vi "Get Transformation Matrix.vi"(9 "Z Axis Rotate Angle":sgl, 10 "Y Axis Rotate Angle":sgl, 11 "Quiver Vector":cluster{"X":sgl, "Y":sgl, "Z":sgl}) -> (1 "Transtlate to Quiver Vertex":sgl[][](array[numeric])=[[1.0, 0.0, 0.0, 0.0], [0.0, 1.0, 0.0, 0.0], [0.0, 0.0, 1.0, 0.0], [0.0, 0.0, 0.0, 1.0]], 2 "Rotate by Z Axis":sgl[][](array[numeric])=[[1.0, 0.0, 0.0, 0.0], [0.0, 1.0, 0.0, 0.0], [0.0, 0.0, 1.0, 0.0], [0.0, 0.0, 0.0, 1.0]], 3 "Rotate by Y Axis":sgl[][](array[numeric])=[[1.0, 0.0, 0.0, 0.0], [0.0, 1.0, 0.0, 0.0], [0.0, 0.0, 1.0, 0.0], [0.0, 0.0, 0.0, 1.0]])   [LabVIEW 2017, in "3D Quiver.lvclass"]
uses:
  <vilib>/Math Plots/3D Math Plots/3D Quiver/3D Quiver/3D Quiver.lvclass
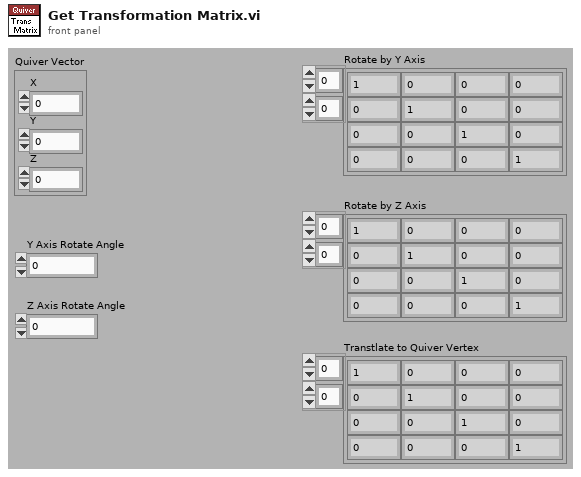
[diagram p1: front panel]
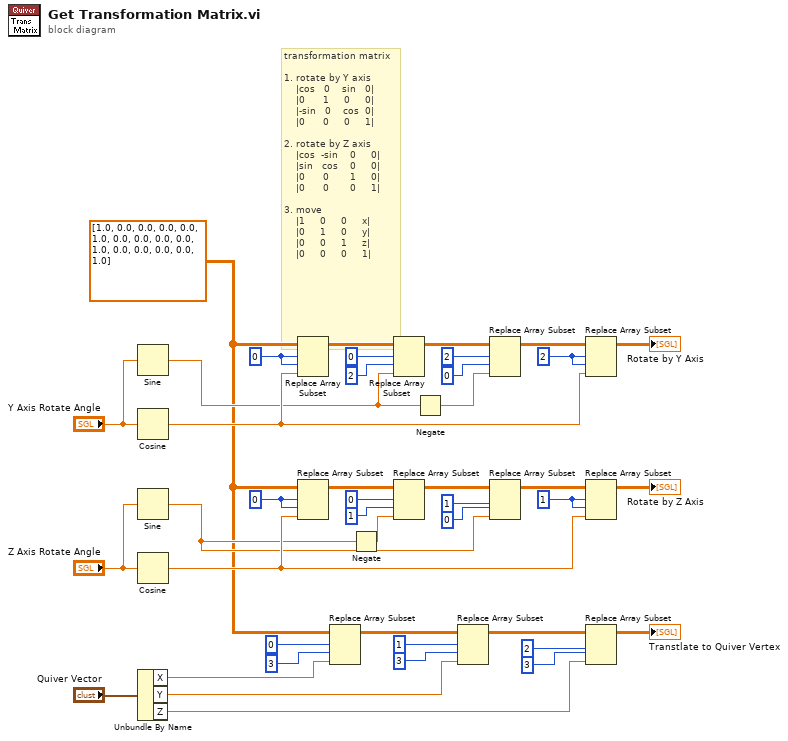
[diagram p0: block diagram]
diagram:
  w9 = sgl[][] [[1.0, 0.0, 0.0, 0.0], [0.0, 1.0, 0.0, 0.0], [0.0, 0.0, 1.0, 0.0], [0.0, 0.0, 0.0, 1.0]] ("Rotate by Y Axis 2")
  w28 = 1 ("index (row)")
  w20 = 0
  w32 = 2 ("index (row)")
  w40 = 0
  # "transformation matrix\n\n1. rotate by Y axis\n    |cos   0    sin   0|\n    |0      1     0     0|\n    |-sin   0    cos  0|\n    |0      0     0     1|\n\n2. rotate by Z axis\n    |cos  -sin    0     0|\n    |sin   cos    0     0|\n    |0      0       1     0|\n    |0      0       0     1|\n\n3. move\n    |1     0     0     x|\n    |0     1     0     y|\n    |0     0     1     z|\n    |0     0     0     1|"
  n1 = Sine(x="Y Axis Rotate Angle") -> (sin(x)=w30:sgl)
  n2 = Cosine(x="Y Axis Rotate Angle") -> (cos(x)=w31:sgl)
  n3 = Sine(x="Z Axis Rotate Angle") -> (sin(x)=w17:sgl)
  n4 = Cosine(x="Z Axis Rotate Angle") -> (cos(x)=w19:sgl)
  n5 = Unbundle By Name("Quiver Vector") -> ("X"=w7:sgl, "Y"=w6:sgl, "Z"=w5:sgl)
  n6 = Replace Array Subset(array=w9, new element=w31, index (row)=w40, index (col)=w40) -> (w39:sgl[][])
  n7 = Replace Array Subset(array=w9, new element=w19, index (row)=w20, index (col)=w20) -> (w21:sgl[][])
  n8 = Replace Array Subset(array=w9, new element=w7, index (row)=0, index (col)=3 ("disabled index (col)")) -> (w15:sgl[][])
  n9 = Negate(x=w17) -> (-x=w18:sgl)
  n10 = Replace Array Subset(array=w39, new element=w30, index (row)=0, index (col)=2 ("disabled index (col)")) -> (w38:sgl[][])
  n11 = Replace Array Subset(array=w21, new element=w18, index (row)=0, index (col)=1 ("disabled index (col)")) -> (w22:sgl[][])
  n12 = Negate(x=w30) -> (-x=w29:sgl)
  n13 = Replace Array Subset(array=w15, new element=w6, index (row)=1, index (col)=3 ("disabled index (col)")) -> (w14:sgl[][])
  n14 = Replace Array Subset(array=w38, new element=w29, index (row)=2, index (col)=0 ("disabled index (col)")) -> (w37:sgl[][])
  n15 = Replace Array Subset(array=w22, new element=w17, index (row)=1, index (col)=0 ("disabled index (col)")) -> (w23:sgl[][])
  n16 = Replace Array Subset(array=w37, new element=w31, index (row)=w32, index (col)=w32) -> (→"Rotate by Y Axis":sgl[][])
  n17 = Replace Array Subset(array=w23, new element=w19, index (row)=w28, index (col)=w28) -> (→"Rotate by Z Axis":sgl[][])
  n18 = Replace Array Subset(array=w14, new element=w5, index (row)=2, index (col)=3 ("disabled index (col)")) -> (→"Transtlate to Quiver Vertex":sgl[][])
